vi "HoloPy_open_holo_file.vi"(6 "imageSize":cluster{"image_size_X":i32, "image_size_Y":i32}, 8 "error in (no error)":errorcluster, 10 "image path":path, 11 "Refnum in":refnum<k35>) -> (0 "error out":errorcluster, 2 "Array":sgl[][](array[numeric]), 3 "Refnum out":refnum<k35>)   [LabVIEW 2025, in "holoTracker.lvlib"]
uses:
  holoTracker.lvlib
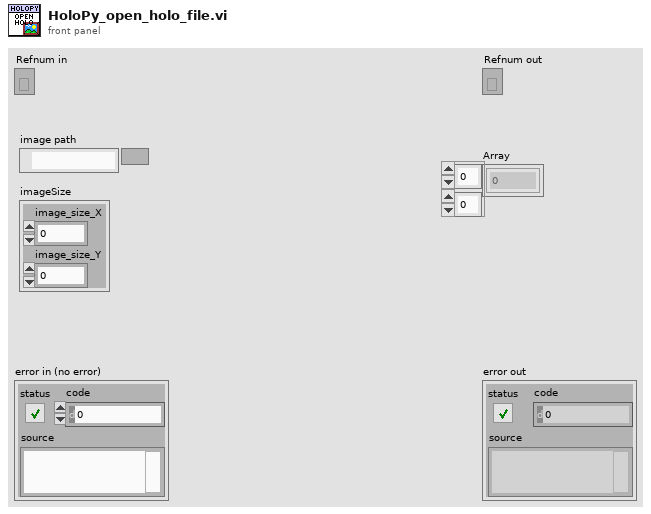
[diagram p1: front panel]
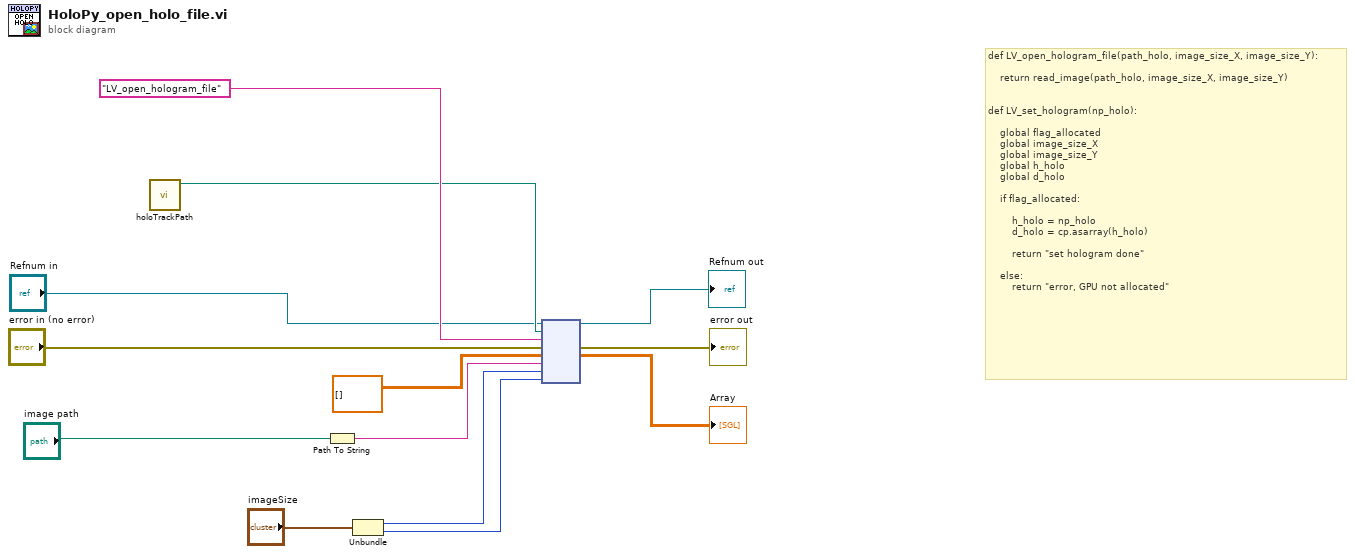
[diagram p0: block diagram]
diagram:
  # "def LV_open_hologram_file(path_holo, image_size_X, image_size_Y):\n\n    return read_image(path_holo, image_size_X, image_size_Y)\n\n\ndef LV_set_hologram(np_holo):\n\n    global flag_allocated\n    global image_size_X \n    global image_size_Y \n    global h_holo\n    global d_holo\n\n    if flag_allocated:\n\n        h_holo = np_holo\n        d_holo = cp.asarray(h_holo)\n\n        return \"set hologram done\"\n    \n    else:\n        return \"error, GPU not allocated\""
  n1 = call "holoTrackPath.vi"() -> ("appended path"=w11:path)  [unwired: 11 in]
  n2 = Path To String(path="image path") -> (string=w7:string)
  n3 = Unbundle("imageSize") -> ("image_size_X"=w3:i32, "image_size_Y"=w2:i32)
  n4 = node("Refnum in", w11, "LV_open_hologram_file" ("function name"), "error in (no error)", sgl[][] [], w7, w3, w2) -> (→"Refnum out":refnum<k35>, →"error out":errorcluster, →"Array":sgl[][])  [unwired: 3 in, 2 out]
